vi "TableControl.vi"(0 "CtlRef":refnum<vi>, 5 "CharIn":i16, 7 "VKey":T1, 9 "ScanCode":i16, 11 "#ofRows":i32) -> (6 "CharOut":i16, 15 "Discard?":bool)   [LabVIEW 2013]
uses:
  <vilib>/event_ctls.llb/eventvkey.ctl
  <vilib>/Utility/miscctls.llb/LVRowAndColumnTypeDef.ctl
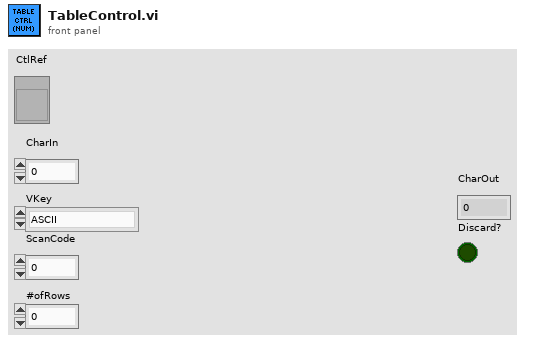
[diagram p1: front panel]
types:
  T1 = typedef "eventvkey.ctl" = enum16{"ASCII", "Enter", "Return", "Shift", "Ctrl", "Alt", "Cmd", "Opt", "Caps", "NumLock", "Clear", "Break", "Up", "Down", "Left", "Right", "Insert", "Delete", "Home", "End", "PageUp", "PageDown", "Escape", "Help", "Pause", "ScrollLock", "F1", "F2", "F3", "F4", "F5", "F6", "F7", "F8", "F9", "F10", "F11", "F12", "F13", "F14", "F15", "F16", "F17", "F18", "F19", "F20", "F21", "F22", "F23", "F24", "Play", "VolumeUp", "VolumeDown", "Mute", "Two Byte Char"}
  T2 = typedef "LVRowAndColumnTypeDef.ctl" = cluster{"Row":i32, "Column":i32}
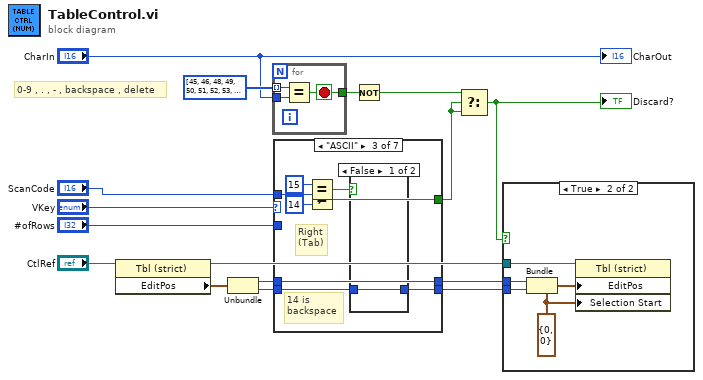
[diagram p0: block diagram]
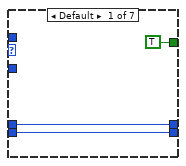
[diagram p3: hidden frame]
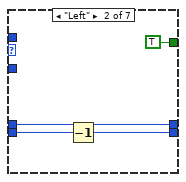
[diagram p4: hidden frame]
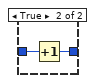
[diagram p5: hidden frame]
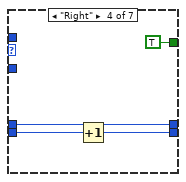
[diagram p6: hidden frame]
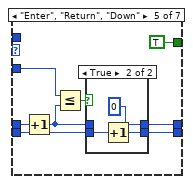
[diagram p7: hidden frame]
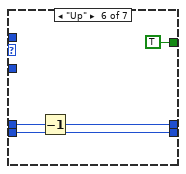
[diagram p9: hidden frame]
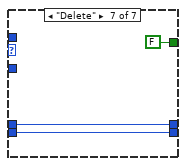
[diagram p10: hidden frame]
diagram:
  # "0-9 , . , - , backspace , delete"
  n1 = property on="Property Node" class="Tbl (strict)"(reference="CtlRef") -> (reference out=w13:refnum<vi>, "EditPos"=w12:T2)  [unwired: 1 in, 1 out]
  n2 = Unbundle(w12) -> ("Row"=w11:i32, "Column"=w10:i32)
  n3 = for {
    tunnel: i16[] [45, 46, 48, 49, 50, 51, 52, 53, 54, 55, 56, 57] -> [w19] mode=indexing
    tunnel: "CharIn" -> [w18]
    tunnel: [w17] -> w4
    stop <- w17 stop-if-true
    n4 = Equal?(x=w19, y=w18) -> (x = y?=w17:bool)
  }
  n5 = case shown="\"ASCII\"" "VKey" {
    tunnel: "ScanCode" -> [_ _ w29 _ _ _ _]
    tunnel: w11 -> [w22 w24 w31 w39 w47 w58 w61]
    tunnel: w10 -> [w21 w26 w32 w41 w46 w57 w60]
    tunnel: [w22 w24 w31 w39 w45 w56 w61] -> w9
    tunnel: [w21 w25 w30 w40 w44 w57 w60] -> w8
    tunnel: "#ofRows" -> [_ _ _ _ w43 _ _]
    tunnel: [TRUE TRUE w27 TRUE TRUE TRUE FALSE] -> w1
    frame Default {
    }
    frame "Left" {
      n6 = Decrement(x=w26) -> (x-1=w25:i32)
    }
    frame "ASCII" {
      # "14 is\nbackspace"
      # "Right\n(Tab)"
      n7 = Equal?(x=i16 15, y=w29) -> (x = y?=w33:bool)
      n8 = Not Equal?(x=w29, y=i16 14 ("x")) -> (x != y?=w27:bool)
      n9 = case shown="False" w33 {
        tunnel: w32 -> [w35 w37]
        tunnel: [w35 w36] -> w30
        frame False {
        }
        frame True {
          n10 = Increment(x=w37) -> (x+1=w36:i32)
        }
      }
    }
    frame "Right" {
      n11 = Increment(x=w41) -> (x+1=w40:i32)
    }
    frame "Enter", "Return", "Down" {
      n12 = Increment(x=w47) -> (x+1=w49:i32)
      n13 = Less Or Equal?(x=w43, y=w49) -> (x <= y?=w48:bool)
      n14 = case shown="True" w48 {
        tunnel: w49 -> [w51 _]
        tunnel: w46 -> [w50 w54]
        tunnel: [w51 0] -> w45
        tunnel: [w50 w53] -> w44
        frame False {
        }
        frame True {
          n15 = Increment(x=w54) -> (x+1=w53:i32)
        }
      }
    }
    frame "Up" {
      n16 = Decrement(x=w58) -> (x-1=w56:i32)
    }
    frame "Delete" {
    }
  }
  n17 = Not(x=w4) -> (.not. x?=w3:bool)
  n18 = Select(t=w3, s=w1, f=w1) -> (s? t:f=w2:bool)
  "Discard?" <- w2
  n19 = case shown="True" w2 {
    tunnel: w13 -> [_ w66]
    tunnel: w9 -> [_ w64]
    tunnel: w8 -> [_ w63]
    frame False {
    }
    frame True {
      w62 = T2 {"Row"=0, "Column"=0} ("Active Cell:Active Cell")
      n20 = Bundle(cluster=w62, "Row"=w64, "Column"=w63) -> (w65:T2)
      n21 = property on="Property Node" class="Tbl (strict)"(reference=w66, "EditPos"=w65, "Selection Start"=w62) -> ()  [unwired: 1 in, 2 out]
    }
  }
  "CharOut" <- "CharIn"
